vi "MQTT_Read_Published_Message.vi"(8 "error in (no error)":errorcluster, 11 "SSL_Connection":T2) -> (0 "error out":errorcluster, 1 "Message":string="MQIsdp", 2 "Topic Name":string="Topic", 3 "SSL_Connection":T2, 4 "MessageType":T1, 5 "Message ID":u16=1 format="%x")   [LabVIEW 2016, in "AWS_IoT.lvlib"]
doc: "This VI reads the last published message at the selected topic. It sends acknowledge information if required by the QoS level.\n\n© 2015 - daq.io, LLC - Peter Adelhardt"
uses:
  AWS_IoT.lvlib
  Controls/SSL_Connection.ctl
  Controls/MessageType.ctl
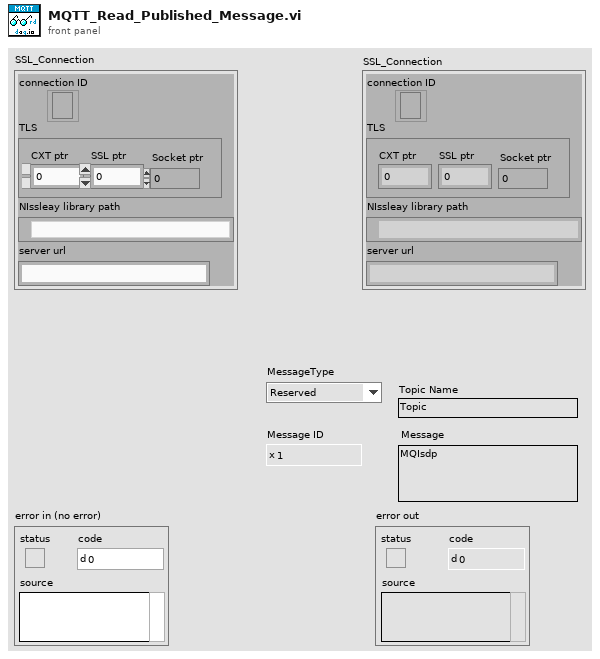
[diagram p1: front panel]
types:
  T1 = typedef "AWS_IoT.lvlib/MessageType.ctl" = enum32{"Reserved", "CONNECT", "CONNACK", "PUBLISH", "PUBACK", "PUBREC", "PUBREL", "PUBCOMP", "SUBSCRIBE", "SUBACK", "UNSUBSCRIBE", "UNSUBACK", "PINGREQ", "PINGRESP", "DISCONNECT", "Reserved2"}
  T2 = typedef "AWS_IoT.lvlib/SSL_Connection.ctl" = cluster{"connection ID":refnum<k5>, "TLS":cluster{"CXT ptr":i32, "SSL ptr":i32, "Socket ptr":i32}, "NIssleay library path":path, "server url":string}
  T3 = typedef "AWS_IoT.lvlib/QoS.ctl" = enum8{"At most once", "At least once", "Exactly once", "Reserved"}
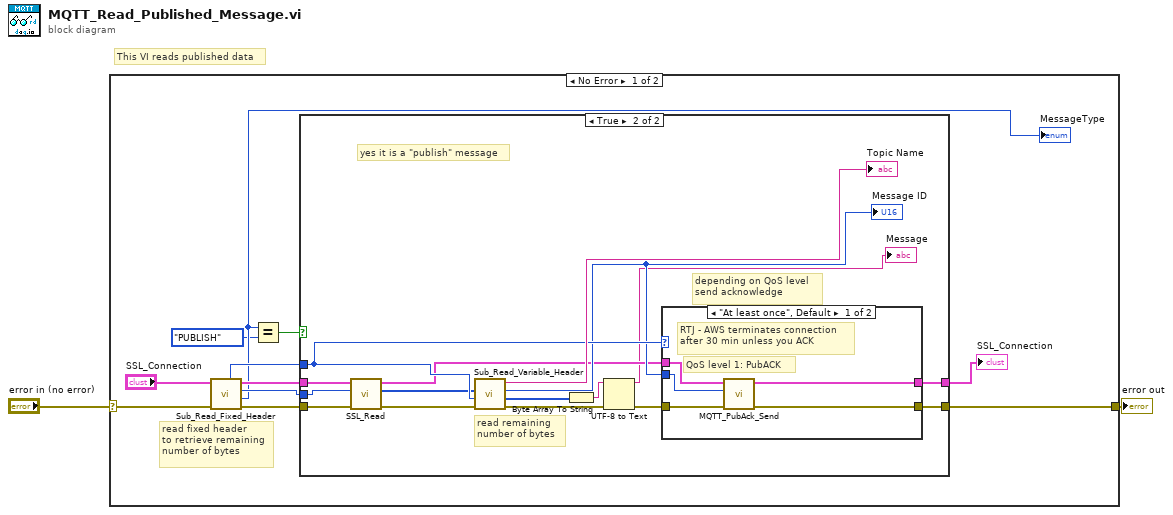
[diagram p0: block diagram]
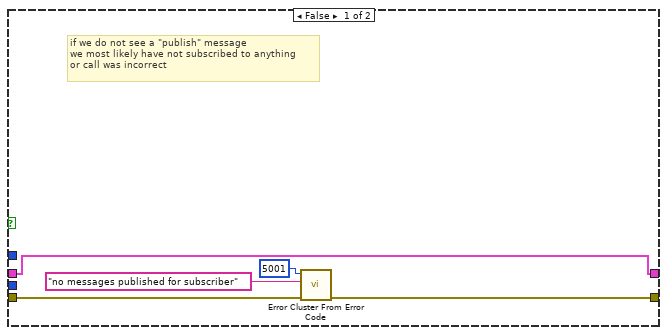
[diagram p2: hidden frame]
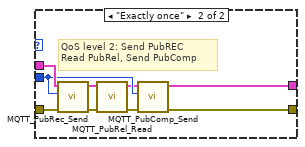
[diagram p3: hidden frame]
diagram:
  # "This VI reads published data"
  n1 = case shown="No Error" "error in (no error)" {
    selector: "error in (no error)" -> [w13 w49]
    tunnel: [w8 w49] -> w1
    frame No Error {
      # "read fixed header \nto retrieve remaining\nnumber of bytes"
      n2 = call "Sub_Read_Fixed_Header.vi"("error in (no error)"=w13, "SSL_Connection"="SSL_Connection") -> ("error out"=w10:errorcluster, "MessageType"=w7:T1, "Remaining Length"=w12:u32, "SSL_Connection"=w11:T2, "QoS Level"=w9:T3)  [unwired: 3 in, 2 out]
      "MessageType" <- w7
      n3 = Equal?(x=w7, y=MessageType."PUBLISH") -> (x = y?=w5:bool)
      n4 = case shown="True" w5 {
        tunnel: w12 -> [_ w33]
        tunnel: w11 -> [w14 w19]
        tunnel: w10 -> [w18 w32]
        tunnel: w9 -> [_ w30]
        tunnel: [w14 w27] -> w3
        tunnel: [w15 w26] -> w8
        frame False {
          # "if we do not see a \"publish\" message\nwe most likely have not subscribed to anything\nor call was incorrect"
          n5 = call <vilib>:"Error Cluster From Error Code.vi"("error in (no error)"=w18, "error message (\"\")"="no messages published for subscriber" ("error message (\"\")"), "error code (0)"=5001) -> ("error out"=w15:errorcluster)  [unwired: 6 in]
        }
        frame True {
          # "yes it is a \"publish\" message"
          # "depending on QoS level\nsend acknowledge"
          # "read remaining\nnumber of bytes"
          n6 = call "SSL_Read.vi"("error in (no error)"=w32, "bytes to read"=w33, "SSL_Connection"=w19) -> ("error out"=w31:errorcluster, "data out"=w20:u8[], "SSL_Connection"=w28:T2)  [unwired: 5 in, 1 out]
          n7 = call "Sub_Read_Variable_Header.vi"("error in (no error)"=w31, "QoS"=w30, "Variable Header"=w20) -> ("error out"=w21:errorcluster, "remaining bytes"=w25:u8[], "Message ID"=w29:u16, "Topic Name"=→"Topic Name":string)  [unwired: 5 in]
          "Message ID" <- w29
          n8 = Byte Array To String(unsigned byte array=w25) -> (string=w24:string)
          n9 = UTF-8 to Text(8:w21, 11:w24) -> (0:w22:errorcluster, 3:→"Message":string)  [unwired: 1 in]
          n10 = case shown="\"At least once\", Default" w30 {
            tunnel: w29 -> [w39 w44]
            tunnel: w22 -> [w38 w48]
            tunnel: w28 -> [w37 w47]
            tunnel: [w36 w46] -> w27
            tunnel: [w35 w45] -> w26
            frame "At least once", Default {
              # "RTJ - AWS terminates connection after 30 min unless you ACK"
              # "QoS level 1: PubACK"
              n11 = call "MQTT_PubAck_Send.vi"("error in (no error)"=w38, "Message ID"=w39, "SSL_Connection"=w37) -> ("error out"=w35:errorcluster, "SSL_Connection"=w36:T2)  [unwired: 6 in, 1 out]
            }
            frame "Exactly once" {
              # "QoS level 2: Send PubREC\nRead PubRel, Send PubComp"
              n12 = call "MQTT_PubRec_Send.vi"("error in (no error)"=w48, "Message ID"=w44, "SSL_Connection"=w47) -> ("error out"=w41:errorcluster, "SSL_Connection"=w40:T2)  [unwired: 6 in, 1 out]
              n13 = call "MQTT_PubRel_Read.vi"("error in (no error)"=w41, "SSL_Connection"=w40) -> ("error out"=w42:errorcluster, "SSL_Connection"=w43:T2)  [unwired: 7 in, 1 out]
              n14 = call "MQTT_PubComp_Send.vi"("error in (no error)"=w42, "Message ID"=w44, "SSL_Connection"=w43) -> ("error out"=w45:errorcluster, "SSL_Connection"=w46:T2)  [unwired: 6 in, 1 out]
            }
          }
        }
      }
      "SSL_Connection" <- w3
    }
    frame Error {
    }
  }
  "error out" <- w1
